vi "libtiff3 close.vi"(7 "error in (no error)":errorcluster, 10 "Handle":i32) -> (0 "error out":errorcluster)   [LabVIEW 2020]
doc: "SciScan 1.0 151216\nClose a file open for reading or writing"
uses:
  DLLs/libtiff3 (32).dll
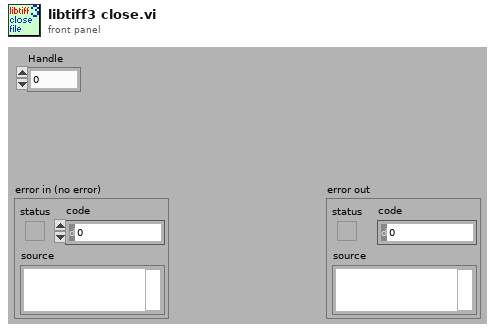
[diagram p1: front panel]
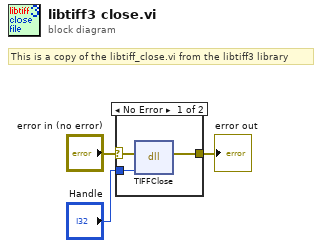
[diagram p0: block diagram]
diagram:
  # "This is a copy of the libtiff_close.vi from the libtiff3 library"
  n1 = case shown="No Error" "error in (no error)" {
    selector: "error in (no error)" -> [w4 w7]
    tunnel: "Handle" -> [w6 _]
    tunnel: [w5 w7] -> w2
    frame No Error {
      n2 = dll-call lib="C:/LocalSVNSCC/Microscope-Software-Commonised-LV/branches/release_3.2_stable_lv2020/support/Libtiff3/DLLs/libtiff3 (32).dll" fn="TIFFClose"(error in=w4, "Handle"=w6) -> (error out=w5:errorcluster)  [unwired: 3 in, 2 out]
    }
    frame Error {
    }
  }
  "error out" <- w2
